vi "Simulation - Cascade and Selector.vi"() -> ()   [LabVIEW 2023]
doc: "This VI demonstrates a cascade and selector control. A compressor, driven by a motor, has a tachometer on it which requires a PID loop to control the speed (the downstream loop). Pressure and flow out of the compressor are fed to individual PID controllers. We want to control the flow, but if the pressure exceeds a specified setpoint, it then becomes the controlled variable. This calls for a \"low select\" function to combine the two upstream controller outputs. The lower of the two outputs then becomes the setpoint for the compressor speed. \n\nRun the VI and note that the PC (pressure controller) and FC (flow controller) turn black when they are selected. Normally, you would leave the pressure setpoint constant. Try making an upward step in flow and notice how the PC takes over control as pressure overshoots. In the real world, a plugged pipe would also cause the pressure loop to take over.\n\nFor simplicity, all variables in this demo are in percent. In a real application, you could normalize all the input and setpoint values to percent before passing them to the PID controllers.\n\nNote that the downstream loop, also known as the inner loop, which is the compressor's speed control, must be faster than the outer loops. A factor of 10 is usually recommended. Otherwise, oscillation is assured. The response speed is simulated through the use of lags."
uses:
  <vilib>/addons/control/pid/pid.llb/PID Lead-Lag (DBL).vi
  <vilib>/addons/control/pid/pid.llb/PID (DBL).vi
  <vilib>/addons/control/pid/NI_PID_pid.lvlib
panel:
  in  "Tab Control":enum32{"Introduction", "Operation"}(tab)
  out "PC":bool
  out "FC":bool
  out "Process Measurements":cluster{dbl, dbl, "output":dbl}(graph)
  out "Speed SP":dbl=45.63008759048858 format="%.2f"
  out "FC N":bool=TRUE
  in  "Flow SP":dbl=70.0
  out "PC N":bool
  in  "Press. SP":dbl=80.0
  in  "Tuning Parameters- Flow":cluster{"Kc":dbl, "Ti":dbl, "Td":dbl}={"Kc"=5.0, "Ti"=0.2, "Td"=0.0} {"Td" format="%#.5g"; "Ti" format="%.2f"; "Kc" format="%.2f"}
  in  "Stop":bool
  in  "Tuning Parameters- Compressor":cluster{"Kc":dbl, "Ti":dbl, "Td":dbl}={"Kc"=1.0, "Ti"=0.1, "Td"=0.005} {"Td" format="%#.5g"; "Ti" format="%.2f"; "Kc" format="%.2f"}
  in  "Tuning Parameters- Pressure":cluster{"Kc":dbl, "Ti":dbl, "Td":dbl}={"Kc"=2.5, "Ti"=0.2, "Td"=0.0} {"Td" format="%#.5g"; "Ti" format="%.2f"; "Kc" format="%.2f"}
  # "Overview: This VI demonstrates a cascade and selector control.  A compressor, driven by a motor, has a tachometer on it which requires a PID loop to control the speed (the downstream loop).  Pressure and flow out of the compressor are fed to individual PID controllers.  We want to control the flow, but if the pressure exceeds a specified setpoint, it then becomes the controlled variable.  This calls for a \"low select\" function to combine the two upstream controller outputs.  The lower of the two outputs then becomes the setpoint for the compressor speed.\n\nRun the VI and note that the PC (pressure controller) and FC (flow controller) turn black when they are selected.  Normally, you would leave the pressure setpoint constant.  Try making an upward step in flow and notice how the PC takes over control as pressure overshoots.  In the real world, a plugged pipe would also cause the pressure loop to take over.\n\nFor simplicity, all variables in this demo are in percent.  In a real application, you could normalize all the input and setpoint values to percent before passing them to the PID controllers.\n\nNote that the downstream loop, also known as the inner loop, which is the compressor's speed control, must be faster than the outer loops.  A factor of 10 is usually recommended.  Otherwise, oscillation is assured.  The response speed is simulated through the use of lags.\nInstructions:\n1. Run the VI.\n2. Verify in the Operation tab how the cascade controllers behave.\n3. Click Stop to stop the VI."
  # "LOW\nSELECT"
  # "TACH"
  # "MOTOR"
  # "COMPRESSOR"
  # "SC"
  # "FT"
  # "PT"
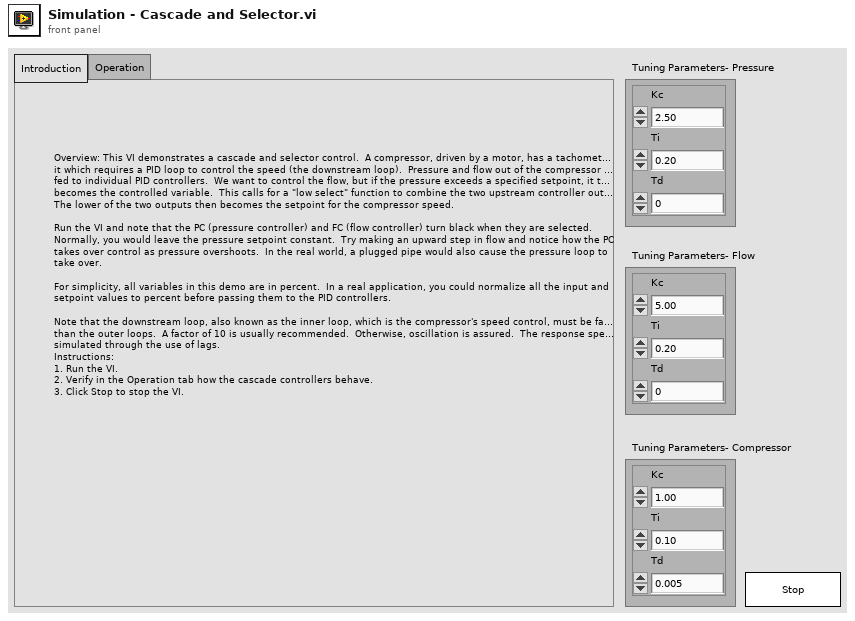
[diagram p1: front panel]
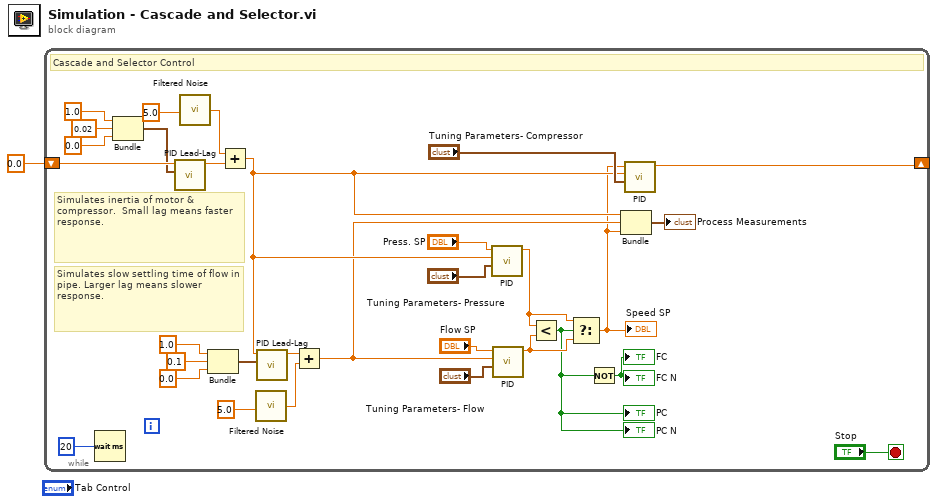
[diagram p0: block diagram]
diagram:
  n1 = while {
    shift-left: 0.0 -> [w30]
    shift-right: [w27] -> _
    stop <- "Stop" stop-if-true
    # "Simulates slow settling time of flow in pipe. Larger lag means slower response."
    # "Simulates inertia of motor & compressor.  Small lag means faster response."
    # "Cascade and Selector Control"
    n2 = Wait (ms)(milliseconds to wait=u32 20) -> ()  [unwired: 1 out]
    n3 = Bundle(1.0, 0.02, 0.0) -> (w9:cluster{dbl, dbl, dbl})  [unwired: 1 in]
    n4 = call-poly <vilib>:"PID Lead-Lag.vi"("tuning parameters"=w9, "input"=w30) -> ("output"=w24:dbl)  [unwired: 6 in, 1 out]
    n5 = call "Filtered Noise.vi"("amplitude: A"=5.0 ("amp2")) -> ("filtered noise"=w21:dbl)
    n6 = Bundle(1.0, 0.1, 0.0) -> (w8:cluster{dbl, dbl, dbl})  [unwired: 1 in]
    n7 = Add(x=w21, y=w24) -> (x+y=w4:dbl)
    n8 = call "Filtered Noise.vi"("amplitude: A"=5.0 ("amp")) -> ("filtered noise"=w23:dbl)
    n9 = call-poly <vilib>:"PID Lead-Lag.vi"("tuning parameters"=w8, "input"=w4) -> ("output"=w28:dbl)  [unwired: 6 in, 1 out]
    n10 = Add(x=w28, y=w23) -> (x+y=w3:dbl)
    n11 = call-poly <vilib>:"PID.vi"("PID gains"="Tuning Parameters- Pressure", "process variable"=w4, "setpoint"="Press. SP") -> ("output"=w26:dbl)  [unwired: 7 in, 1 out]
    n12 = call-poly <vilib>:"PID.vi"("PID gains"="Tuning Parameters- Flow", "process variable"=w3, "setpoint"="Flow SP") -> ("output"=w25:dbl)  [unwired: 7 in, 1 out]
    n13 = Less?(x=w26, y=w25) -> (x < y?=w5:bool)
    "PC N" <- w5
    "PC" <- w5
    n14 = Select(t=w26, s=w5, f=w25) -> (s? t:f=w2:dbl)
    "Speed SP" <- w2
    n15 = Not(x=w5) -> (.not. x?=→"FC N" →"FC":bool)
    n16 = Bundle(w4, w3, "output"=w2) -> (→"Process Measurements":cluster{dbl, dbl, "output":dbl})  [unwired: 1 in]
    n17 = call-poly <vilib>:"PID.vi"("PID gains"="Tuning Parameters- Compressor", "process variable"=w4, "setpoint"=w2) -> ("output"=w27:dbl)  [unwired: 7 in, 1 out]
  }
